vi "Build Tx UDP Engine Configuration.vi"(0 "section ref in":T8=18446744073709551615 format="%.0x", 5 "board properties":T6 {"portConfig" items=["FDX_SINGLE", "FDX_REDUNDANT"]; "portSpeed" items=["FDX_100MBIT", "FDX_10MBIT", "FDX_AUTO_100MBIT", "FDX_AUTO_10MBIT", "FDX_AUTO_ERROR", "FDX_1000MBIT"]}, 9 "port properties":T5, 11 "error in":errorcluster) -> (4 "section ref out":T8 format="%.0x", 6 "boardId":u32, 8 "portId":u32, 10 "VL configurations":T7(array[cluster]) {"VL Config"."NetSelect" items=["FDX_TX_FRAME_DLY_A"=0, "FDX_TX_FRAME_DLY_B"=1, "FDX_TX_FRAME_BOTH "=3, "FDX_TX_FRAME_ONLY_A"=4, "FDX_TX_FRAME_ONLY_B "=5]; "VL Config"."interfaceID" format="%.0b"}, 14 "comm port payload":T4(array[cluster]) {"Parameters"."encoding" items=["BNR", "BCD", "Discrete", "Signed_32", "Signed_64", "Float_32", "Float_64", "Opaque"]}, 15 "error out":errorcluster)   [LabVIEW 2020, in "AIM ARINC 664 Scripting.lvlib"]
uses:
  AIM ARINC 664 Scripting.lvlib
  <vilib>/NI VeriStand/Custom Device API/Custom Device Item Ref.ctl
  <instrlib>/AIM GmbH/_AIM 664/_controls/comm_config_vl_tx.ctl
  <instrlib>/AIM GmbH/_AIM 664/_controls/comm_udp_tx.ctl
  Import/_typedefs/board_setup.ctl
  Import/_typedefs/port_setup.ctl
  Shared/Encoding (Arinc664).ctl
  Import/_typedefs/frame_parameter_definition.ctl
  Constants.vi
  <vilib>/NI VeriStand/Custom Device API/Get Item Property (String).vi
  <instrlib>/AIM GmbH/_AIM 664/AIM664LV.lvlib
  <vilib>/NI VeriStand/Custom Device API/Custom Device API.lvlib
  Import/AIM ARINC 664 Import.lvlib
panel:
  in  "Cluster":cluster{"VL Config":T1, "CommPort Config":T2[]} {"VL Config"."NetSelect" items=["FDX_TX_FRAME_DLY_A"=0, "FDX_TX_FRAME_DLY_B"=1, "FDX_TX_FRAME_BOTH "=3, "FDX_TX_FRAME_ONLY_A"=4, "FDX_TX_FRAME_ONLY_B "=5]; "VL Config"."interfaceID" format="%.0b"}
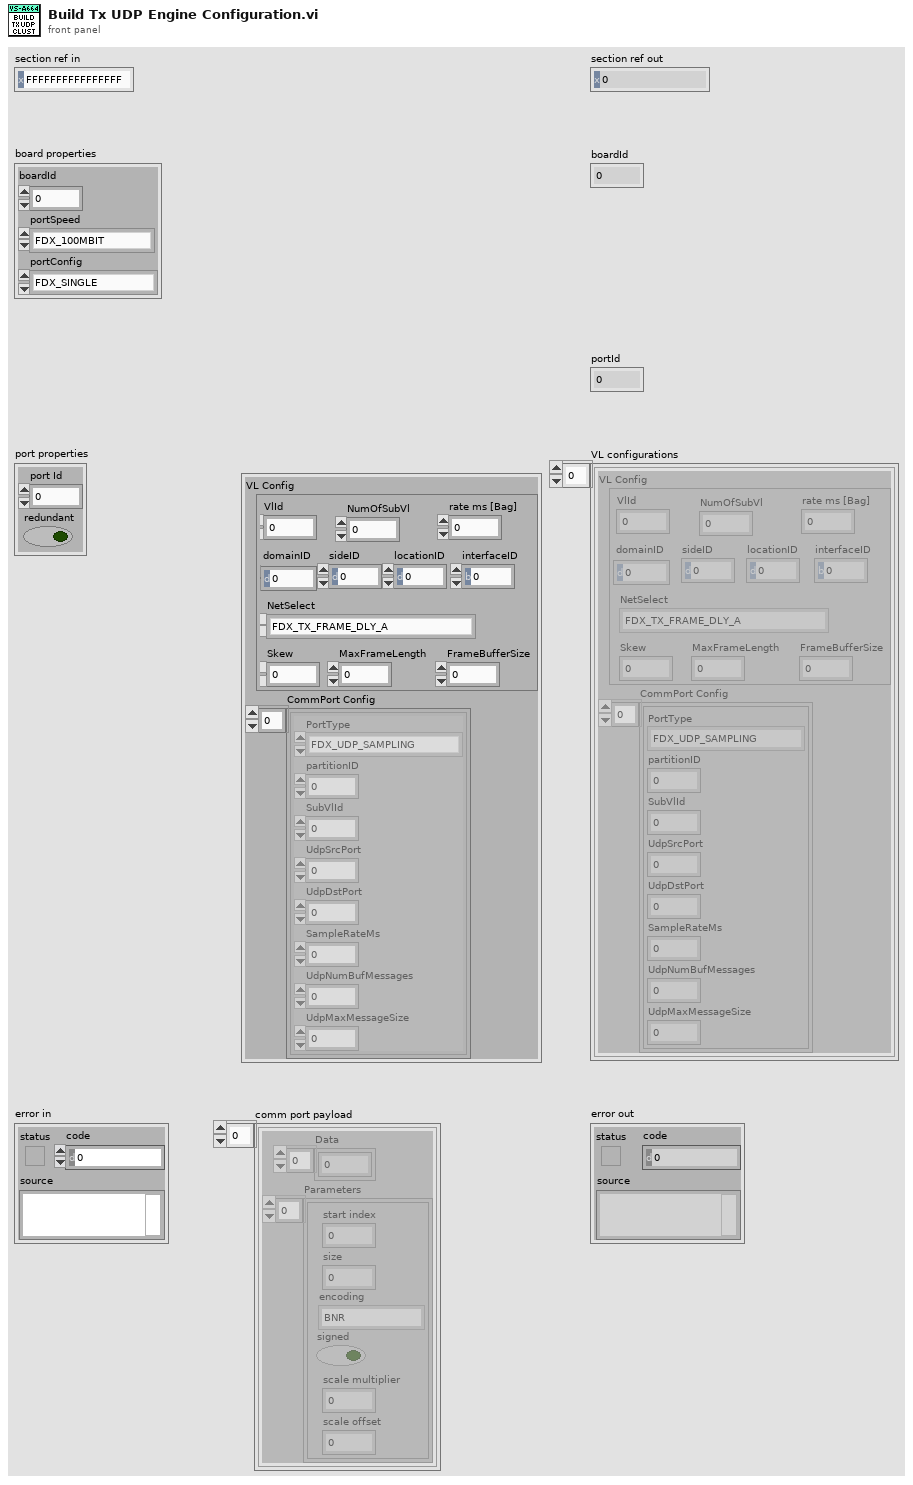
[diagram p1: front panel]
types:
  T1 = typedef "AIM664LV.lvlib/comm_config_vl_tx.ctl" = cluster{"VlId":u16, "NumOfSubVl":u16, "rate ms [Bag]":u32, "domainID":u8, "sideID":u8, "locationID":u8, "interfaceID":u8, "NetSelect":u32, "Skew":u32, "MaxFrameLength":u32, "FrameBufferSize":u32}
  T2 = typedef "AIM664LV.lvlib/comm_udp_tx.ctl" = cluster{"PortType":enum16{"FDX_UDP_SAMPLING", "FDX_UDP_QUEUING"}, "partitionID":u8, "SubVlId":u8, "UdpSrcPort":u16, "UdpDstPort":u16, "SampleRateMs":dbl, "UdpNumBufMessages":u32, "UdpMaxMessageSize":u32}
  T3 = typedef "Encoding (Arinc664).ctl" = u16
  T4 = cluster{"Data":u8[], "Parameters":cluster{"start index":i32, "size":i32, "encoding":T3, "signed":bool, "scale multiplier":dbl, "scale offset":dbl}[]}[]
  T5 = typedef "AIM ARINC 664 Import.lvlib/port_setup.ctl" = cluster{"port Id":u32, "redundant":bool}
  T6 = typedef "AIM ARINC 664 Import.lvlib/board_setup.ctl" = cluster{"boardId":u32, "portSpeed":u32, "portConfig":u32}
  T7 = cluster{"VL Config":T1, "CommPort Config":T2[]}[]
  T8 = typedef "Custom Device API.lvlib/Custom Device Item Ref.ctl" = u64
  T9 = typedef "AIM ARINC 664 Import.lvlib/frame_parameter_definition.ctl" = cluster{"start index":i32, "size":i32, "encoding":T3, "signed":bool, "scale multiplier":dbl, "scale offset":dbl}
  T10 = cluster{"Data":u8[], "Parameters":cluster{"start index":i32, "size":i32, "encoding":T3, "signed":bool, "scale multiplier":dbl, "scale offset":dbl}[]}
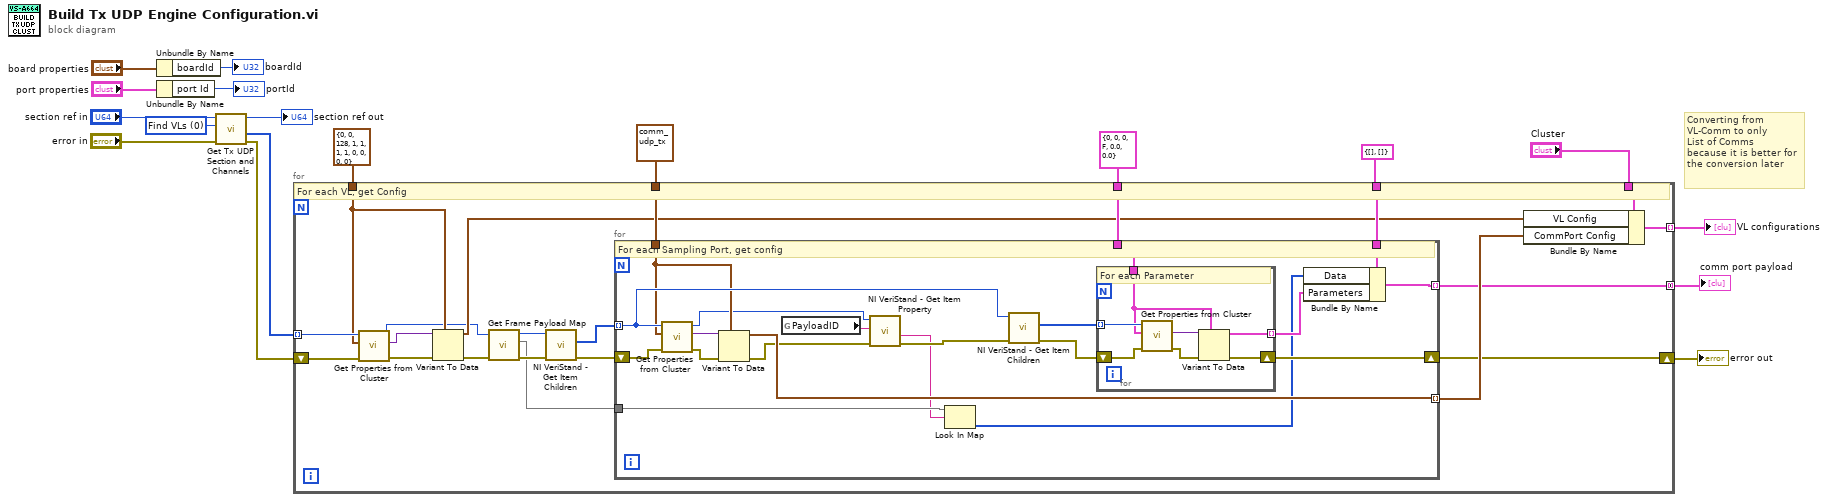
[diagram p0: block diagram]
diagram:
  w13 = u16 0 items=["Find VLs", "Find Parameters"] ("Option")
  # "Converting from \nVL-Comm to only\nList of Comms\nbecause it is better for\nthe conversion later"
  n1 = Unbundle By Name("board properties") -> ("boardId"=→"boardId":u32)
  n2 = Unbundle By Name("port properties") -> ("port Id"=→"portId":u32)
  n3 = call "Get Tx UDP Section and Channels.vi"("error in"="error in", "option"=w13, "custom device ref in"="section ref in") -> ("error out"=w9:errorcluster, "Tx UDP channel refs out"=w4:T8[], "custom device ref out"=→"section ref out":T8)  [unwired: 3 in, 3 out]
  n4 = for {
    tunnel: [w32] -> w16 mode=indexing
    tunnel: w4 -> [w39] mode=indexing
    tunnel: T1 {"VlId"=0, "NumOfSubVl"=0, "rate ms [Bag]"=128, "domainID"=1, "sideID"=1, "locationID"=1, "interfaceID"=1, "NetSelect"=0, "Skew"=0, "MaxFrameLength"=0, "FrameBufferSize"=0} ("CommPort Config") -> [w37]
    shift-right: [w26] -> w5
    shift-left: w9 -> [w38]
    tunnel: T2 {"PortType"=enum."FDX_UDP_SAMPLING", "partitionID"=0, "SubVlId"=1, "UdpSrcPort"=0, "UdpDstPort"=0, "SampleRateMs"=128.0, "UdpNumBufMessages"=0, "UdpMaxMessageSize"=0} ("commPort config") -> [w31]
    tunnel: T9 {"start index"=0, "size"=0, "encoding"=0, "signed"=FALSE, "scale multiplier"=0.0, "scale offset"=0.0} ("Parameter 2") -> [w29]
    tunnel: [w27] -> w2 mode=concatenating
    tunnel: T10 {"Data"=[], "Parameters"=[]} ("Data and Parameters") -> [w28]
    tunnel: "Cluster" -> [w24]
    # "For each VL, get Config"
    n5 = call "Get Properties from Cluster.vi"("error in"=w38, "Variant Cluster"=w37, "custom device ref in"=w39) -> ("error out"=w35:errorcluster, "data"=w36:variant, "custom device ref out"=w23:T8)  [unwired: 5 in, 1 out]
    n6 = Variant To Data(error in=w35, type=w37, Variant=w36) -> (data=w25:T1, error out=w22:errorcluster)
    n7 = call "Get Frame Payload Map.vi"("error in"=w22, "custom device ref in"=w23) -> ("error out"=w20:errorcluster, "Payload Map"=w19:map{string, u8[]}, "custom device ref out"=w21:T8)  [unwired: 7 in]
    n8 = call <vilib>:"NI VeriStand - Get Item Children.vi"("error in (no error)"=w20, "Item Ref in"=w21) -> ("error out"=w33:errorcluster, "Child Refs"=w34:T8[])  [unwired: 6 in, 2 out]
    n9 = for {
      tunnel: w34 -> [w57] mode=indexing
      shift-right: [w47] -> w26
      shift-left: w33 -> [w50]
      tunnel: w31 -> [w56]
      tunnel: [w55] -> w30 mode=indexing
      tunnel: w29 -> [w54]
      tunnel: w28 -> [w53]
      tunnel: [w51] -> w27 mode=indexing
      tunnel: w19 -> [w42]
      # "For each Sampling Port, get config"
      n10 = call "Get Properties from Cluster.vi"("error in"=w50, "Variant Cluster"=w56, "custom device ref in"=w57) -> ("error out"=w59:errorcluster, "data"=w58:variant, "custom device ref out"=w43:T8)  [unwired: 5 in, 1 out]
      n11 = Variant To Data(error in=w59, type=w56, Variant=w58) -> (data=w55:T2, error out=w45:errorcluster)
      n12 = global read "Constants.vi" "PayloadID"() -> (w46:string)
      n13 = call-poly <vilib>:"NI VeriStand - Get Item Property.vi"("error in (no error)"=w45, "Property Name"=w46, "Item Ref in"=w43) -> ("error out"=w44:errorcluster, "Value"=w41:string)  [unwired: 5 in, 2 out]
      n14 = Look In Map(map=w42, key=w41) -> (value=w40:u8[])  [unwired: 1 in, 1 out]
      n15 = call <vilib>:"NI VeriStand - Get Item Children.vi"("error in (no error)"=w44, "Item Ref in"=w57) -> ("error out"=w48:errorcluster, "Child Refs"=w49:T8[])  [unwired: 6 in, 2 out]
      n16 = for {
        tunnel: w49 -> [w64] mode=indexing
        shift-right: [w60] -> w47
        shift-left: w48 -> [w61]
        tunnel: w54 -> [w63]
        tunnel: [w62] -> w52 mode=indexing
        # "For each Parameter"
        n17 = call "Get Properties from Cluster.vi"("error in"=w61, "Variant Cluster"=w63, "custom device ref in"=w64) -> ("error out"=w65:errorcluster, "data"=w66:variant)  [unwired: 5 in, 2 out]
        n18 = Variant To Data(error in=w65, type=w63, Variant=w66) -> (data=w62:T9, error out=w60:errorcluster)
      }
      n19 = Bundle By Name(cluster=w53, "Data"=w40, "Parameters"=w52) -> (w51:T10)
    }
    n20 = Bundle By Name(cluster=w24, "VL Config"=w25, "CommPort Config"=w30) -> (w32:cluster{"VL Config":T1, "CommPort Config":T2[]})
  }
  "error out" <- w5
  "VL configurations" <- w16
  "comm port payload" <- w2
